vi "AAL Resample Filter Prototype Design.vi"(8 "error in (no error)":errorcluster, 9 "alias free":bool, 10 "normalized bandwidth":dbl=0.4536 format="%.4f", 11 "A stop [dB]":dbl=72.0 format="%.2f") -> (0 "error out":errorcluster, 2 "taps":i32, 3 "filter prototype":cluster{"coefficients":dbl[], "factor":i32}={"coefficients"=[], "factor"=1} {"coefficients" format="%.2f"})   [LabVIEW 2024, in "NI_AALPro.lvlib"]
doc: "Design a filter prototype for arbitrary resampling."
uses:
  NI_AALPro.lvlib
panel:
  in  "maximum decimation factor (auto)":i32
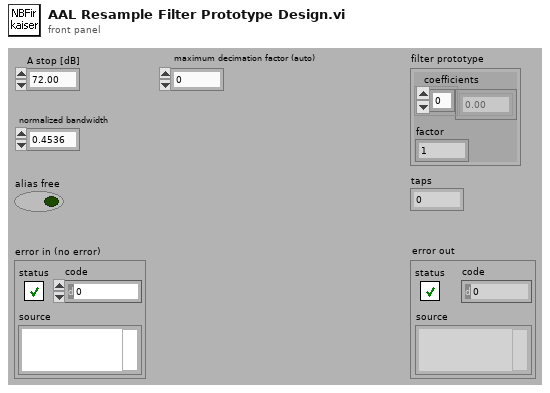
[diagram p1: front panel]
types:
  T1 = cluster{"maximum decimation factor (auto)":i32, "alias free":bool, "A stop [dB]":dbl, "timing jitter":enum32{"Interpolation", "Rounding"}, "normalized bandwidth":dbl}
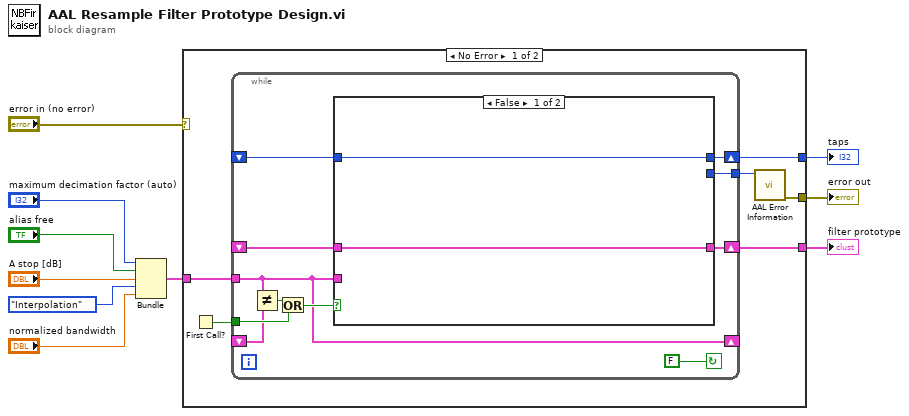
[diagram p0: block diagram]
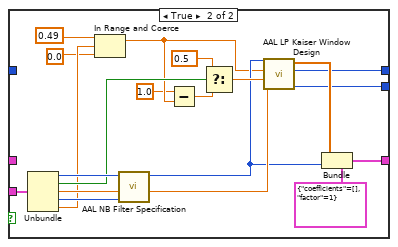
[diagram p2: hidden frame]
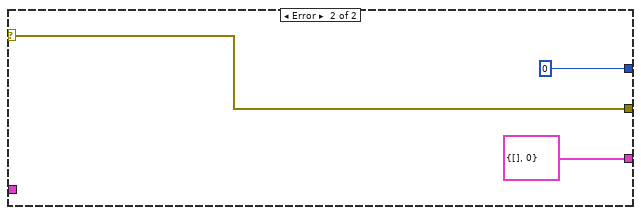
[diagram p3: hidden frame]
diagram:
  n1 = Bundle("maximum decimation factor (auto)"="maximum decimation factor (auto)", "alias free"="alias free", "A stop [dB]"="A stop [dB]", "timing jitter"=enum32{"Interpolation", "Rounding"}."Interpolation", "normalized bandwidth"="normalized bandwidth") -> (w10:T1)  [unwired: 1 in]
  n2 = case shown="No Error" "error in (no error)" {
    selector: "error in (no error)" -> [_ w52]
    tunnel: w10 -> [w16 _]
    tunnel: [w13 0 ("taps")] -> w3
    tunnel: [w12 w52] -> w2
    tunnel: [w11 cluster{"coefficients":dbl[], "factor":i32} {"coefficients"=[], "factor"=0} ("filter prototype")] -> w1
    frame No Error {
      n3 = First Call?() -> (First Call?: T/F=w15:bool)
      n4 = while {
        shift-right: [w27] -> w11
        shift-left: _ -> [w21]
        shift-right: [w18] -> _
        shift-left: _ -> [w19]
        tunnel: w16 -> [w18]
        shift-right: [w25] -> w13
        shift-left: _ -> [w20]
        tunnel: w15 -> [w24]
        tunnel: [w17] -> w14
        stop <- FALSE continue-if-true
        n5 = Not Equal?(x=w18, y=w19) -> (x != y?=w23:bool)
        n6 = Or(x=w23, y=w24) -> (x .or. y?=w22:bool)
        n7 = case shown="False" w22 {
          tunnel: [w30 w46] -> w25
          tunnel: [w29 w49] -> w27
          tunnel: w18 -> [_ w48]
          tunnel: w20 -> [w30 _]
          tunnel: w21 -> [w29 _]
          tunnel: [0 ("error") w37] -> w17
          frame False {
          }
          frame True {
            n8 = Unbundle(w48) -> ("maximum decimation factor (auto)"=w43:i32, "alias free"=w39:bool, "A stop [dB]"=w42:dbl, "timing jitter"=w41:enum32{"Interpolation", "Rounding"}, "normalized bandwidth"=w35:dbl)
            n9 = In Range and Coerce(upper limit=0.49, x=w35, lower limit=0.0) -> (coerced(x)=w33:dbl)  [unwired: 1 out]
            n10 = call "AAL NB Filter Specification.vi"("timing jitter"=w41, "stop band attenuation"=w42, "maximum decimation factor"=w43) -> ("A stop [dB]"=w40:dbl, "decimation factor"=w38:i32)  [unwired: 7 in]
            n11 = Subtract(x=1.0, y=w33) -> (x-y=w31:dbl)
            n12 = Select(t=0.5, s=w39, f=w31) -> (s? t:f=w45:dbl)
            n13 = call "AAL LP Kaiser Window Design.vi"("A stop [dB]"=w40, "stopband"=w45, "passband"=w33, "fs"=w38) -> ("error"=w37:i32, "taps"=w46:i32, "filter coefficients"=w47:dbl[])  [unwired: 5 in]
            n14 = Bundle(cluster=cluster{"coefficients":dbl[], "factor":i32} {"coefficients"=[], "factor"=1} ("filter prototype"), "coefficients"=w47, "factor"=w38) -> (w49:cluster{"coefficients":dbl[], "factor":i32})
          }
        }
      }
      n15 = call "AAL Error Information.vi"("error code"=w14) -> ("error out"=w12:errorcluster)  [unwired: 10 in]
    }
    frame Error {
    }
  }
  "error out" <- w2
  "taps" <- w3
  "filter prototype" <- w1
